vi "Configure Resolution.vi"(0 "VISA resource name":refnum<visa-resource-name>, 5 "Motor ID (0)":u8, 7 "Resolution (2048)":u8(ring)=1 items=["2048"=1, "1024"=2, "683"=3, "512"=4], 11 "error in (no error)":errorcluster) -> (4 "VISA resource name out":refnum<visa-resource-name>, 15 "error out":errorcluster)   [LabVIEW 2016, in "Dynamixel Motor.lvlib"]
doc: "Sets the resolution of the motor position."
uses:
  Dynamixel Motor.lvlib
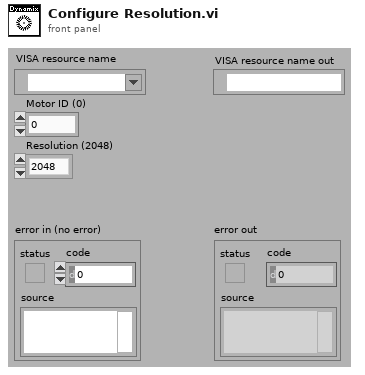
[diagram p1: front panel]
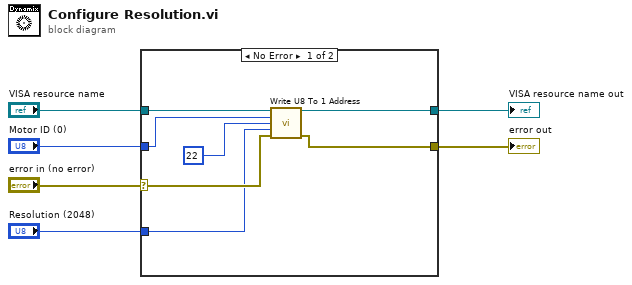
[diagram p0: block diagram]
diagram:
  n1 = case shown="No Error" "error in (no error)" {
    selector: "error in (no error)" -> [w10 w15]
    tunnel: "VISA resource name" -> [w13 w14]
    tunnel: [w12 w14] -> w5
    tunnel: [w11 w15] -> w4
    tunnel: "Motor ID (0)" -> [w7 _]
    tunnel: "Resolution (2048)" -> [w8 _]
    frame No Error {
      n2 = call "Write U8 To 1 Address.vi"("VISA resource name"=w13, "Motor ID (0)"=w7, "Address number (0)"=u8 22 ("Address"), "Parameter (0)"=w8, "error in (no error)"=w10) -> ("VISA resource name out"=w12:refnum<visa-resource-name>, "error out"=w11:errorcluster)  [unwired: 9 in]
    }
    frame Error {
    }
  }
  "VISA resource name out" <- w5
  "error out" <- w4
